vi "Jeffress_model_v002.vi"() -> ()   [LabVIEW 2019]
panel:
  out "new picture":picture
  out "Left - Right":dbl
  out "Elapsed time 1":dbl caption="Get Start Time (s)"
  out "Elapsed time 2":dbl caption="Get Start Time (s)"
  in  "stop":bool
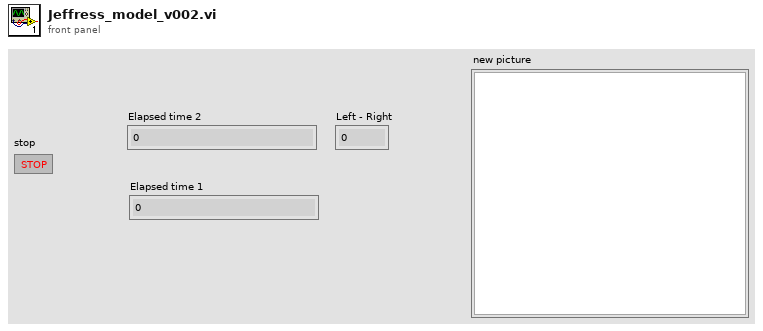
[diagram p1: front panel]
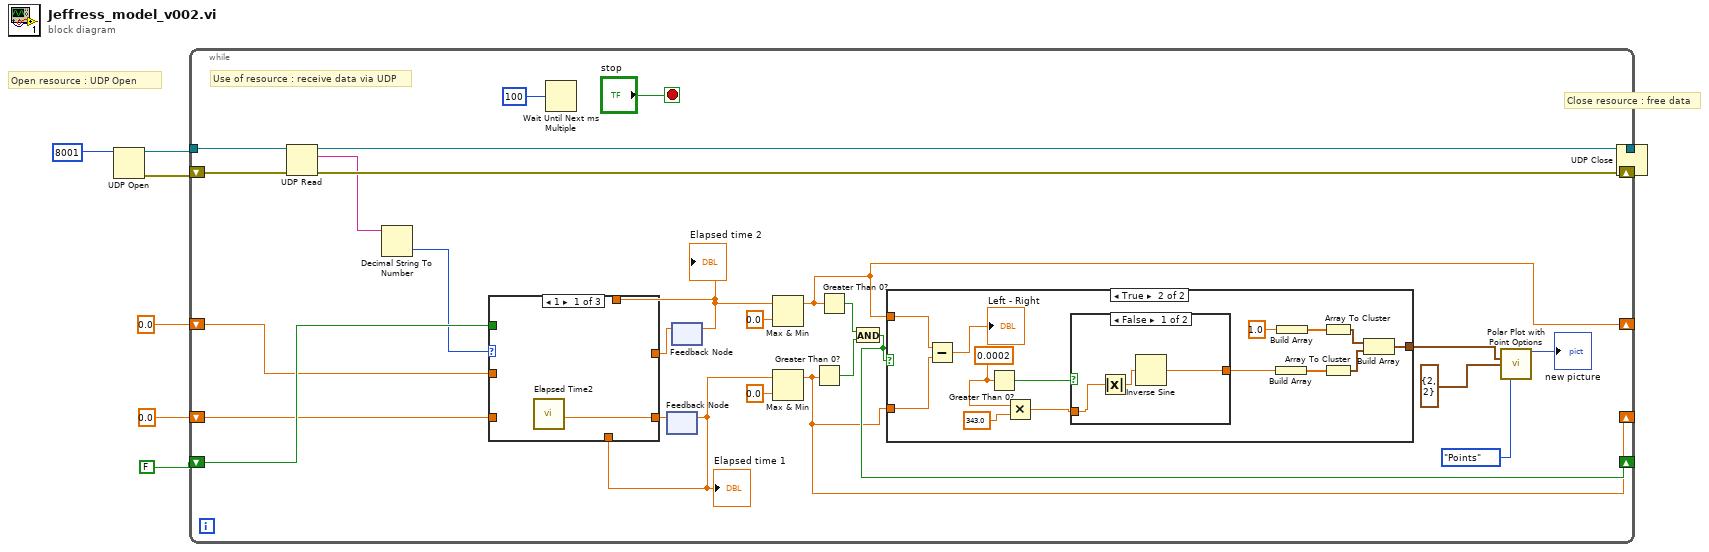
[diagram p0: block diagram]
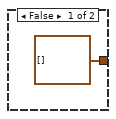
[diagram p2: hidden frame]
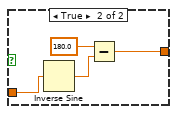
[diagram p3: hidden frame]
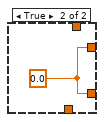
[diagram p5: hidden frame]
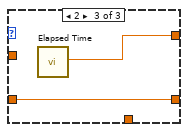
[diagram p6: hidden frame]
diagram:
  # "Close resource : free data"
  # "Open resource : UDP Open"
  n1 = UDP Open(11:u16 8001) -> (port=w6:refnum<k16>, 0:w8:errorcluster)  [unwired: 4 in, 1 out]
  n2 = while {
    tunnel: w6 -> [w30]
    tunnel: [w29] -> w5
    shift-right: [w32] -> w7
    shift-left: w8 -> [w31]
    shift-right: [w24] -> _
    shift-left: FALSE -> [w23]
    shift-right: [w20] -> _
    shift-left: 0.0 -> [w19]
    shift-right: [w22] -> _
    shift-left: 0.0 -> [w21]
    stop <- "stop" stop-if-true
    # "Use of resource : receive data via UDP"
    n3 = UDP Read(connection ID=w30, 8:w31) -> (data out=w9:string, error out=w32:errorcluster, 3:w29:refnum<k16>)  [unwired: 2 in, 2 out]
    n4 = Decimal String To Number(string=w9) -> (number=w10:i32)  [unwired: 2 in, 1 out]
    n5 = Wait Until Next ms Multiple(millisecond multiple=u32 100) -> ()  [unwired: 1 out]
    n6 = feedback #1() -> (w15:dbl)  [unwired: 1 in]
    "Elapsed time 1" <- w15
    n7 = feedback #2() -> (w17:dbl)  [unwired: 1 in]
    "Elapsed time 2" <- w17
    n8 = case shown="1" w10 {
      tunnel: [w57 w61 w68] -> w16
      tunnel: [w58 w62 w67] -> w18
      tunnel: w23 -> [_ w63 _]
      tunnel: w21 -> [_ _ w68]
      tunnel: w19 -> [w58 _ _]
      tunnel: w17 -> [_ w60 _]
      tunnel: w15 -> [_ w59 _]
      frame 1 {
        n9 = call "Elapsed Time2"() -> ("Elapsed Time (s)"=w57:dbl)  [unwired: 12 in, 7 out]
      }
      frame Default {
        n10 = case shown="False" w63 {
          tunnel: [w65 w66] -> w62
          tunnel: [w64 w66] -> w61
          tunnel: w60 -> [w65 _]
          tunnel: w59 -> [w64 _]
          frame False {
          }
          frame True {
            w66 = 0.0
          }
        }
      }
      frame 2 {
        n11 = call "Elapsed Time"() -> ("Elapsed Time (s)"=w67:dbl)  [unwired: 12 in, 7 out]
      }
    }
    n12 = feedback-in #1(w16) -> ()
    n13 = feedback-in #2(w18) -> ()
    n14 = Max & Min(x=w17, y=0.0) -> (max(x,y)=w20:dbl)  [unwired: 1 out]
    n15 = Max & Min(x=w15, y=0.0) -> (max(x,y)=w22:dbl)  [unwired: 1 out]
    n16 = Greater Than 0?(x=w22) -> (x > 0?=w25:bool)
    n17 = Greater Than 0?(x=w20) -> (x > 0?=w26:bool)
    n18 = And(x=w26, y=w25) -> (x .and. y?=w24:bool)
    n19 = case shown="True" w24 {
      tunnel: w20 -> [_ w48]
      tunnel: w22 -> [_ w49]
      tunnel: [cluster{"[0]":dbl, "[1]":dbl}[] [] w40] -> w14
      frame False {
      }
      frame True {
        w36 = 0.0002
        n20 = Subtract(x=w48, y=w49) -> (x-y=→"Left - Right":dbl)
        n21 = Greater Than 0?(x=w36) -> (x > 0?=w47:bool)
        n22 = Multiply(x=w36, y=343.0) -> (x*y=w37:dbl)
        n23 = case shown="False" w47 {
          tunnel: w37 -> [w50 w56]
          tunnel: [w52 w53] -> w43
          frame False {
            n24 = Absolute Value(x=w50) -> (abs(x)=w51:dbl)
            n25 = Inverse Sine(1:w51) -> (0:w52:dbl)
          }
          frame True {
            n26 = Inverse Sine(1:w56) -> (0:w55:dbl)
            n27 = Subtract(x=180.0, y=w55) -> (x-y=w53:dbl)
          }
        }
        n28 = Build Array(w43) -> (w44:dbl[])
        n29 = Build Array(1.0 ("element")) -> (w45:dbl[])
        n30 = Array To Cluster(array=w45) -> (cluster=w41:cluster{"[0]":dbl, "[1]":dbl})
        n31 = Array To Cluster(array=w44) -> (cluster=w42:cluster{"[0]":dbl, "[1]":dbl})
        n32 = Build Array(w41, w42) -> (w40:cluster{"[0]":dbl, "[1]":dbl}[])
      }
    }
    n33 = call <vilib>:"Polar Plot with Point Options.vi"("data array [mag, phase (deg)]"=w14, "top left point(0, 0)"=cluster{"x":i16, "y":i16} {"x"=2, "y"=2}, "Lines/Points"=enum16{"Lines", "Points"}."Points") -> ("new picture"=→"new picture":picture)  [unwired: 12 in]
  }
  n34 = UDP Close(connection ID=w5, 8:w7) -> ()  [unwired: 2 out]
